vi "Initialize Python Optimization (On-Grid).vi"(8 "error in":errorcluster, 11 "On-Grid in":refnum<class "On-Grid.lvclass">) -> (0 "error out":errorcluster, 3 "On-Grid out":refnum<class "On-Grid.lvclass">)   [LabVIEW 2018, in "On-Grid Actor.lvlib" / "On-Grid.lvclass"]
uses:
  On-Grid.lvclass
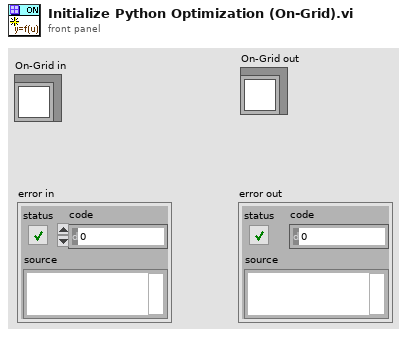
[diagram p1: front panel]
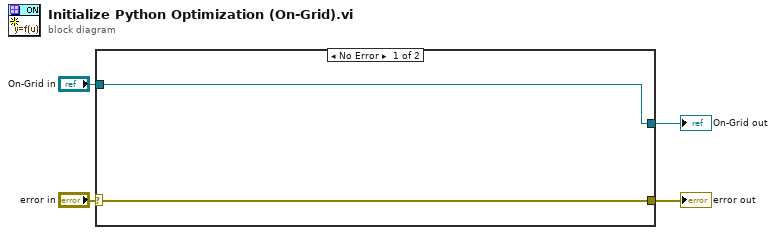
[diagram p0: block diagram]
diagram:
  n1 = case shown="No Error" "error in" {
    selector: "error in" -> [w6 w7]
    tunnel: [w6 w7] -> w4
    tunnel: "On-Grid in" -> [w5 w8]
    tunnel: [w5 w8] -> w1
    frame No Error {
    }
    frame Error {
    }
  }
  "error out" <- w4
  "On-Grid out" <- w1
